vi "CheckForLabVIEW_IDE.vi"() -> (0 "LabVIEW IDE":bool)   [LabVIEW 2013, in "VITesterUtilities.lvlib"]
uses:
  Libraries/VITesterUtilities.lvlib
  JKI Reuse/X in Y (Variant)__jki_lib_array -- VI Tester.vi
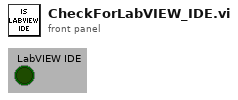
[diagram p1: front panel]
types:
  T1 = enum32{"invalid app kind", "Development System", "Run Time System", "Student Edition", "Embedded LabVIEW", "Evaluation", "Custom"}[]
  T2 = enum32{"invalid app kind", "Development System", "Run Time System", "Student Edition", "Embedded LabVIEW", "Evaluation", "Custom"}
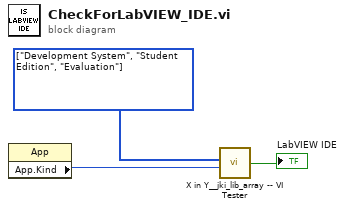
[diagram p0: block diagram]
diagram:
  w3 = T1 [enum."Development System", enum."Student Edition", enum."Evaluation"] items=["invalid app kind", "Development System", "Run Time System", "Student Edition", "Embedded LabVIEW", "Evaluation", "Custom"]
  n1 = property class="App"() -> ("App.Kind"=w2:T2)  [unwired: 2 in, 2 out]
  n2 = call-poly "X in Y__jki_lib_array -- VI Tester.vi"("array"=w3, "element"=w2) -> ("element in array?"=→"LabVIEW IDE":bool)  [unwired: 5 in]
